vi "DB parameterized query example.vi"(8 "error in (no error)":errorcluster, 11 "File Location":T1=-2 items=["Currently Writing"=-3, "Labview Files"=-2, "Mars Data Processing Factility"=-1, "Local Cache "=0, "Old Storage"=1, "Storage"=2]) -> (0 "error out":errorcluster, 3 "BP Array":T2[](array[typedef]) {"File Location" items=["Currently Writing"=-3, "Labview Files"=-2, "Mars Data Processing Factility"=-1, "Local Cache "=0, "Old Storage"=1, "Storage"=2]})   [LabVIEW 2012]
uses:
  Batch Processor/bp_cluster.ctl
  Private/File_location.ctl
  <vilib>/addons/database/Auxilliary.llb/DB Tools Parameter Info.ctl
  <vilib>/addons/database/Auxilliary.llb/DB Tools DataTypes.ctl
  <vilib>/addons/database/Auxilliary.llb/DB Tools Parameter Dir.ctl
  <vilib>/addons/database/Command.llb/Cmd Set Parameter Value (C).vi
  <vilib>/addons/database/Command.llb/Cmd Execute.vi
  <vilib>/addons/database/Recordset.llb/Rec Fetch Recordset Data (CR).vi
  <vilib>/addons/database/Recordset.llb/Rec Destroy - Command.vi
  <vilib>/addons/database/Command.llb/Cmd Delete.vi
  <vilib>/addons/database/_DB Variant To Data/Database Variant To Data.xnode
  <vilib>/addons/database/NI_Database_API.lvlib
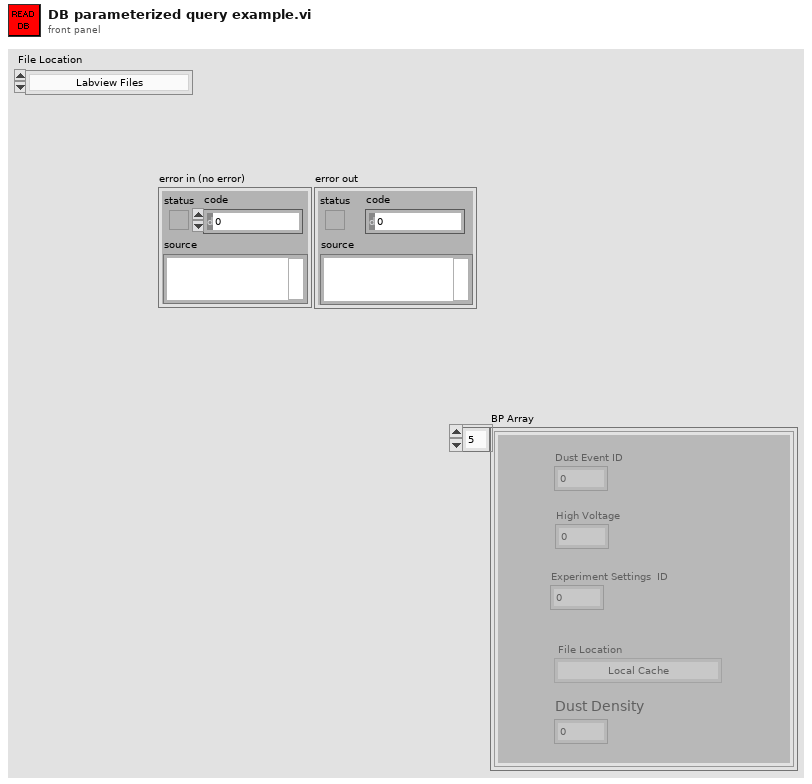
[diagram p1: front panel]
types:
  T1 = typedef "File_location.ctl" = i8
  T2 = typedef "bp_cluster.ctl" = cluster{"Dust Event ID":i64, "High Voltage":sgl, "Experiment Settings  ID":i64, "File Location":T1, "Dust Density":dbl}
  T3 = typedef "NI_Database_API.lvlib/DB Tools Parameter Info.ctl" = cluster{"parameter name":string, "type":T4, "direction":T5, "value":variant}
  T4 = typedef "NI_Database_API.lvlib/DB Tools DataTypes.ctl" = enum16{"String", "Long (I32)", "Single (SGL)", "Double (DBL)", "Date/Time", "Binary"}
  T5 = typedef "NI_Database_API.lvlib/DB Tools Parameter Dir.ctl" = enum32{"Input", "Output", "Input/Output", "Return Value"}
  T6 = typedef "NI_Database_API.lvlib/Conn ObjectReference.ctl" = refnum<k1>
  T7 = typedef "NI_Database_API.lvlib/Cmd ObjectReference.ctl" = refnum<k1>
  T8 = typedef "NI_Database_API.lvlib/Cmd-Rec Object Reference.ctl" = refnum<k1>
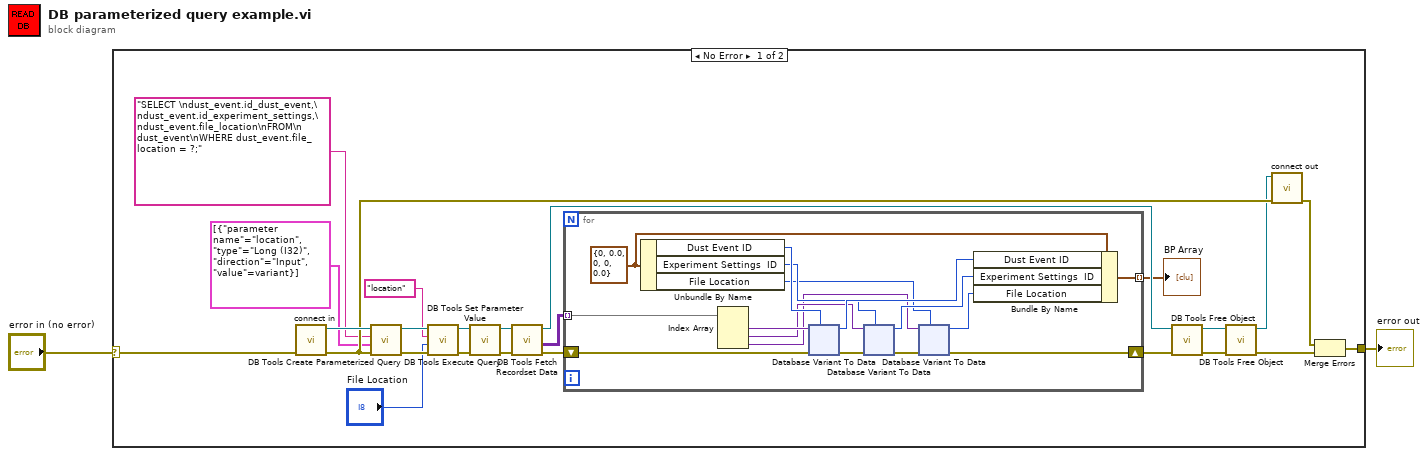
[diagram p0: block diagram]
diagram:
  n1 = case shown="No Error" "error in (no error)" {
    selector: "error in (no error)" -> [w7 w139]
    tunnel: [w18 w139] -> w1
    frame No Error {
      n2 = call "connect in.vi"("error in (no error)"=w7) -> ("error out"=w16:errorcluster, "Database Connection"=w17:T6)  [unwired: 6 in, 1 out]
      n3 = call <vilib>:"DB Tools Create Parameterized Query.vi"("error in (no error)"=w16, "parameters"=T3[] [{"parameter name"="location", "type"=enum."Long (I32)", "direction"=enum."Input", "value"=variant}], "SQL query"="SELECT \ndust_event.id_dust_event,\ndust_event.id_experiment_settings,\ndust_event.file_location\nFROM\n    dust_event\nWHERE dust_event.file_location = ?;" ("string"), "connection reference"=w17) -> ("error out"=w14:errorcluster, "command reference"=w15:T7)  [unwired: 3 in, 1 out]
      n4 = call-poly <vilib>:"DB Tools Set Parameter Value.vi"("error in (no error)"=w14, "value"="File Location", "parameter index"="location" ("parameter name"), "command reference"=w15) -> ("error out"=w8:errorcluster, "command reference out"=w9:T7)  [unwired: 4 in]
      n5 = call-poly <vilib>:"DB Tools Execute Query.vi"("error in (no error)"=w8, "command reference"=w9) -> ("error out"=w25:errorcluster, "command-recordset reference"=w26:T8)  [unwired: 6 in]
      n6 = call-poly <vilib>:"DB Tools Fetch Recordset Data.vi"("error in (no error)"=w25, "command-recordset reference"=w26) -> ("error out"=w23:errorcluster, "recordset data"=w21:variant[][], "command-recordset reference out"=w24:T8)  [unwired: 3 in]
      n7 = for {
        tunnel: w21 -> [w42] mode=indexing
        shift-right: [w27] -> w22
        shift-left: w23 -> [w41]
        tunnel: [w39] -> w20 mode=indexing
        w36 = T2 {"Dust Event ID"=0, "High Voltage"=0.0, "Experiment Settings  ID"=0, "File Location"=0, "Dust Density"=0.0} ("Batch Processing Cluster")
        n8 = Unbundle By Name(w36) -> ("Dust Event ID"=w38:i64, "Experiment Settings  ID"=w35:i64, "File Location"=w30:T1)
        n9 = Index Array(array=w42) -> (element #1=w40:variant, element #2=w32:variant, element #3=w31:variant)  [unwired: 3 in]
        n10 = xnode "Database Variant To Data"("database variant"=w40, "error in"=w41, "type"=w38) -> ("data"=w37:i64, "error out"=w33:errorcluster)
        n11 = xnode "Database Variant To Data"("database variant"=w32, "error in"=w33, "type"=w35) -> ("data"=w34:i64, "error out"=w28:errorcluster)
        n12 = xnode "Database Variant To Data"("database variant"=w31, "error in (no error)"=w28, "type"=w30) -> ("data"=w29:T1, "error out"=w27:errorcluster)
        n13 = Bundle By Name(cluster=w36, "Dust Event ID"=w37, "Experiment Settings  ID"=w34, "File Location"=w29) -> (w39:T2)
      }
      "BP Array" <- w20
      n14 = call-poly <vilib>:"DB Tools Free Object.vi"("error in (no error)"=w22, "command-recordset reference"=w24) -> ("error out"=w11:errorcluster, "command reference"=w4:T7)  [unwired: 8 in]
      n15 = call-poly <vilib>:"DB Tools Free Object.vi"("error in (no error)"=w11, "command reference"=w4) -> ("error out"=w10:errorcluster, "connection reference"=w12:T6)  [unwired: 8 in]
      n16 = call "connect out.vi"("error in (no error)"=w16, "connection reference"=w12) -> ("error out"=w19:errorcluster)  [unwired: 9 in]
      n17 = Merge Errors(w19, w10) -> (w18:errorcluster)
    }
    frame Error {
    }
  }
  "error out" <- w1
